vi "Moving Graph.vi"() -> ()   [LabVIEW 2014]
uses:
  <vilib>/measure/NI_MABase.lvlib
panel:
  in  "Knob":dbl(knob) scale=0.0..10.0
  in  "Boolean":bool
  out "Waveform Graph 2":dbl[](graph)
  out "Waveform Graph":waveform(dbl)(graph)
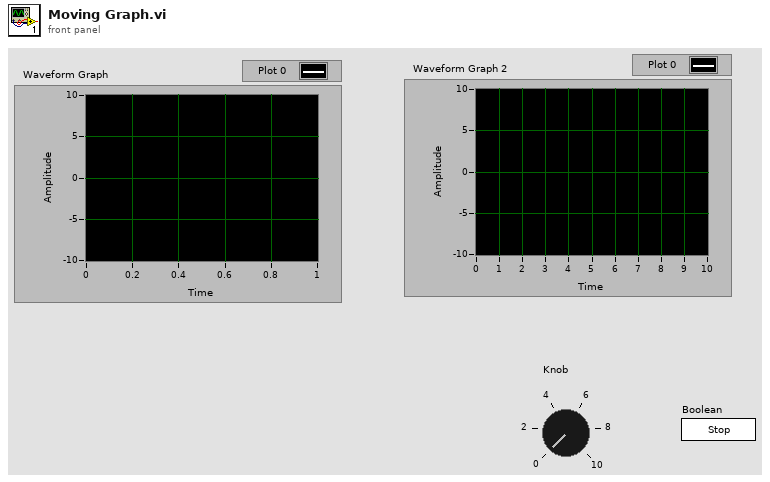
[diagram p1: front panel]
types:
  T1 = enum16{"Sine Wave", "Triangle Wave", "Square Wave", "Sawtooth Wave"}
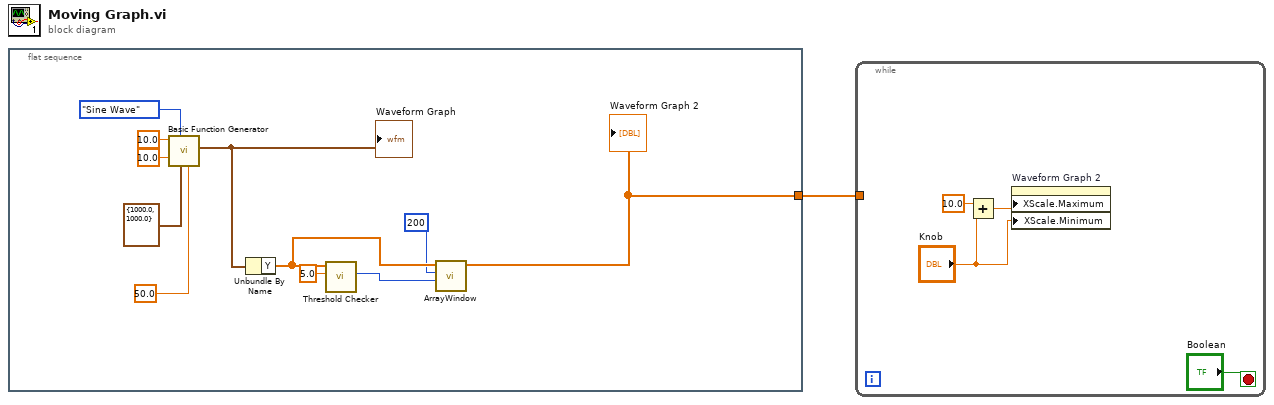
[diagram p0: block diagram]
diagram:
  n1 = flat-sequence {
    tunnel: [w2] -> w1
    frame #0 {
      n2 = call <vilib>:"Basic Function Generator.vi"("square wave duty cycle (%)"=50.0, "sampling info"=cluster{"Fs":dbl, "#s":dbl} {"Fs"=1000.0, "#s"=1000.0}, "signal type"=T1."Sine Wave", "amplitude"=10.0, "frequency"=10.0) -> ("signal out"=w7:waveform(dbl))  [unwired: 4 in, 2 out]
      "Waveform Graph" <- w7
      n3 = Unbundle By Name(w7) -> ("Y"=w4:dbl[])
      n4 = call "Threshold Checker.vi"("Threshold"=5.0, "Data"=w4) -> ("Index of Value = to or exceeding threshold"=w5:i32)  [unwired: 7 in, 2 out]
      n5 = call "ArrayWindow.VI"("Index"=w5, "Total amount of Pts"=200, "Input Y-values"=w4) -> ("Output Array"=w2:dbl[])  [unwired: 8 in]
      "Waveform Graph 2" <- w2
    }
  }
  n6 = while {
    tunnel: w1 -> [_]
    stop <- "Boolean" stop-if-true
    n7 = Add(x=10.0, y="Knob") -> (x+y=w14:dbl)
    n8 = property on="Waveform Graph 2" class="WFGraph (strict)"("XScale.Maximum"=w14, "XScale.Minimum"="Knob") -> ()  [unwired: 2 in, 2 out]
  }
